vi "Time2ModJulianDate.vi"(4 "Time of Propagation (UTC)  2":timestamp=timestamp(3487974106 s since 1904-01-01) format="%^<%H:%M:%S\n%x>T") -> (0 "ModifiedJulian":dbl format="%#_17g", 1 "PartOfDay":dbl, 2 "JDay":dbl, 3 "JD":dbl format="%#.15g")   [LabVIEW 2013]
panel:
  out "Offset in [hr]":dbl
  out "Local-time":timestamp
  out "UTC-time":timestamp
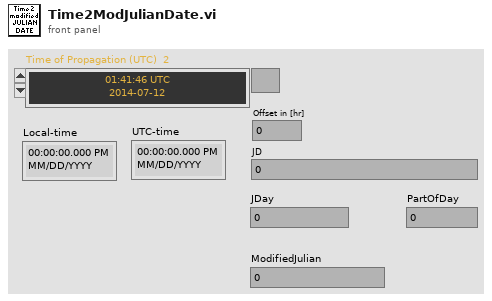
[diagram p1: front panel]
types:
  T1 = cluster{"second":i32, "minute":i32, "hour":i32, "day of month":i32, "month":i32, "year":i32, "day of week":i32, "day of year":i32, "is DST":i32}
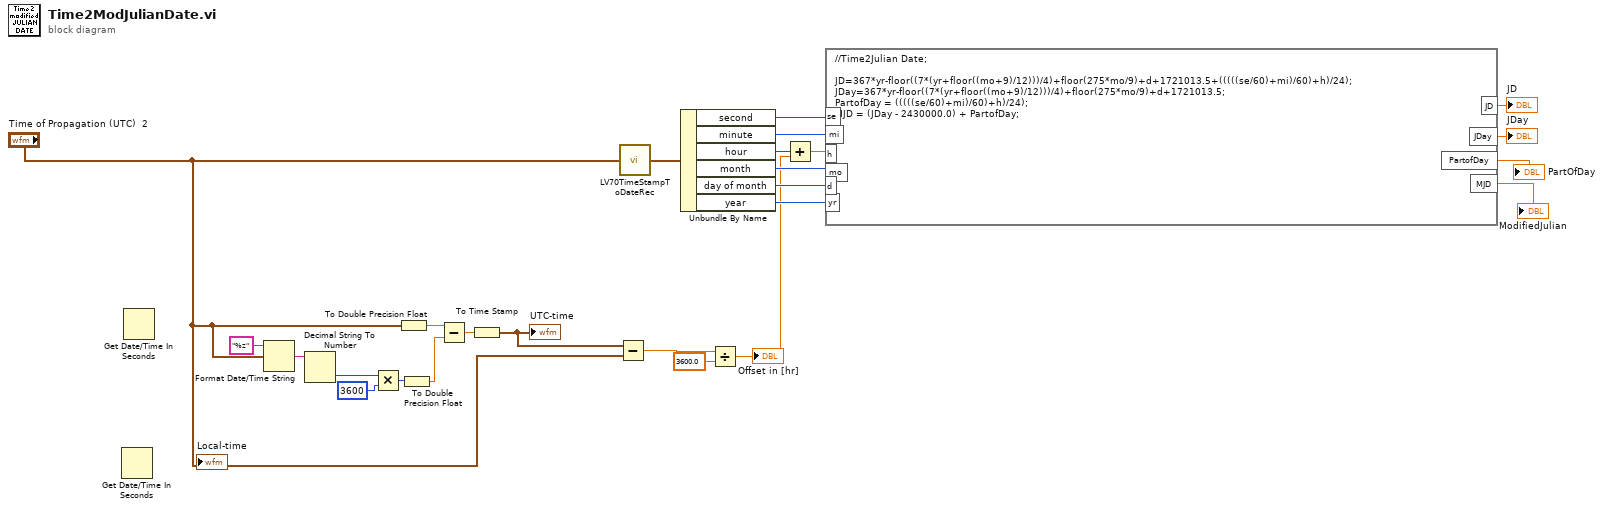
[diagram p0: block diagram]
diagram:
  n1 = Get Date/Time In Seconds() -> ()  [unwired: 1 out]
  n2 = Get Date/Time In Seconds() -> ()  [unwired: 1 out]
  n3 = Format Date/Time String(time format string (%c)="%z", seconds (now)="Time of Propagation (UTC)  2") -> (date/time string=w10:string)  [unwired: 1 out]
  n4 = Decimal String To Number(string=w10) -> (number=w9:i32)  [unwired: 3 out]
  n5 = Multiply(x=w9, y=3600) -> (x*y=w14:i32)
  n6 = To Double Precision Float(number="Time of Propagation (UTC)  2") -> (double precision float=w13:dbl)
  n7 = To Double Precision Float(number=w14) -> (double precision float=w12:dbl)
  n8 = Subtract(x=w13, y=w12) -> (x-y=w11:dbl)
  n9 = To Time Stamp(1:w11) -> (0:w8:timestamp)
  "UTC-time" <- w8
  n10 = Subtract(x=w8, y="Time of Propagation (UTC)  2") -> (x-y=w7:dbl)
  n11 = call <vilib>:"LV70TimeStampToDateRec.vi"("time stamp"="Time of Propagation (UTC)  2") -> ("date time rec"=w24:T1)
  n12 = Unbundle By Name(w24) -> ("second"=w23:i32, "minute"=w22:i32, "hour"=w18:i32, "month"=w21:i32, "day of month"=w20:i32, "year"=w19:i32)
  n13 = Divide(x=w7, y=3600.0) -> (x/y=w4:dbl)
  "Offset in [hr]" <- w4
  n14 = Add(x=w18, y=w4) -> (x+y=w17:dbl)
  n15 = formula code="//Time2Julian Date;\n\nJD=367*yr-floor((7*(yr+floor((mo+9)/12)))/4)+floor(275*mo/9)+d+1721013.5+(((((se/60)+mi)/60)+h)/24);\nJDay=367*yr-floor((7*(yr+floor((mo+9)/12)))/4)+floor(275*mo/9)+d+1721013.5;\nPartofDay = (((((se/60)+mi)/60)+h)/24);\nMJD = (JDay - 2430000.0) + PartofDay;"("yr"=w19, "mo"=w21, "d"=w20, "h"=w17, "mi"=w22, "se"=w23) -> ("JD"=→"JD":dbl, "JDay"=→"JDay":dbl, "PartofDay"=→"PartOfDay":dbl, "MJD"=→"ModifiedJulian":dbl)
  "Local-time" <- "Time of Propagation (UTC)  2"
